vi "Queues vs Local Variables.vi"() -> ()   [LabVIEW 2009]
panel:
  in  "Durée de la boucle (ms)":u16(ring)=50 items=["La même que la boucle productrice"=50, "Vitesse maximale"=0, "2 fois la boucle productrice"=25, "1/2 de la boucle productrice"=100, "1/20 de la boucle productrice"=1000]
  out "Nb de points manqués":i32
  in  "Durée de la boucle (ms)":u16(ring)=50 items=["La même que la boucle productrice"=50, "Vitesse maximale"=0, "2 fois la boucle productrice"=25, "1/2 de la boucle productrice"=100, "1/20 de la boucle productrice"=1000]
  out "Nb d'éléments dans\nla file d'attente":i32(slide) caption="Nb d'éléments dans la file d'attente" scale=0.0..1000.0
  out "Nb de points générés par la boucle productrice":i32
  in  "Stop":bool
  out "Boucle consommatrice de variable locale":dbl(graph)
  out "Boucle consommatrice de file d'attente":dbl(graph)=-9.510565162951542
  out "Boucle productrice":dbl(graph)
  # "Boucle productrice"
  # "Durée de la boucle = 50 ms"
  # "Boucle consommatrice de variable locale"
  # "Boucle consommatrice de file d'attente"
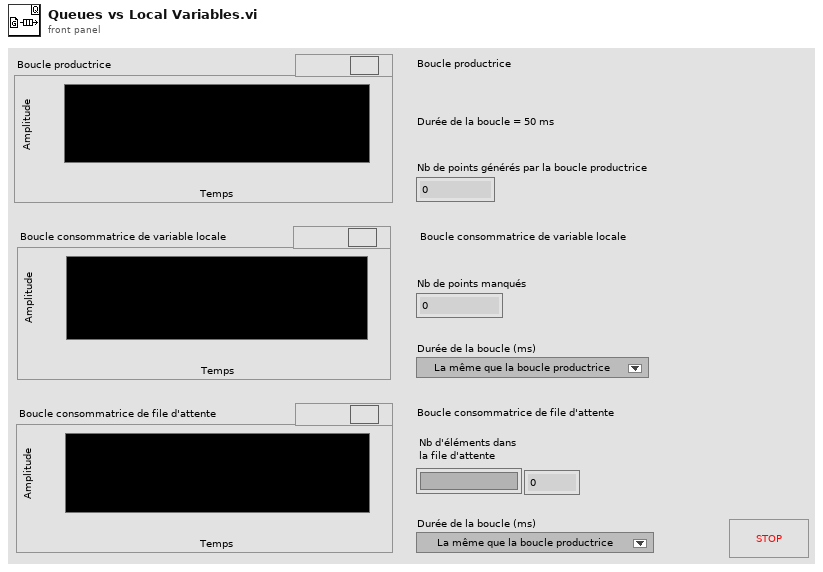
[diagram p1: front panel]
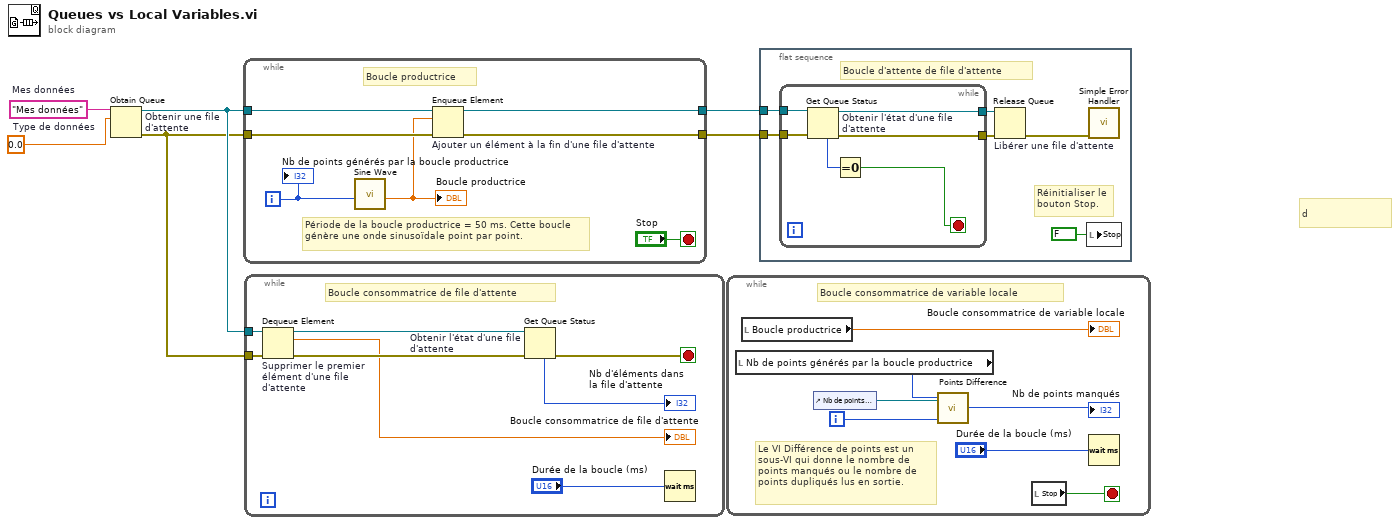
[diagram p0: block diagram]
diagram:
  w5 = "Mes données"  # Mes données
  w6 = 0.0  # Type de données
  # "d"
  n1 = Obtain Queue "Obtenir une file d'attente"(name (unnamed)=w5, element data type=w6) -> (queue out=w4:refnum<queue>, error out=w1:errorcluster)  [unwired: 3 in, 1 out]
  n2 = while {
    tunnel: w4 -> [w11]
    tunnel: w1 -> [w10]
    tunnel: [w8] -> w3
    tunnel: [w7] -> w2
    i -> [w12]
    stop <- "Stop" stop-if-true
    # "Période de la boucle productrice = 50 ms. Cette boucle génère une onde sinusoïdale point par point."
    # "Boucle productrice"
    n3 = call "Sine Wave.vi"("Numérique"=w12) -> ("Signal sinusoïdal"=w9:dbl)  [unwired: 6 out]
    "Boucle productrice" <- w9
    n4 = Enqueue Element "Ajouter un élément à la fin d'une file d'attente"(queue=w11, element=w9, error in (no error)=w10) -> (queue out=w7:refnum<queue>, error out=w8:errorcluster)  [unwired: 2 out]
    "Nb de points générés par la boucle productrice" <- w12
  }
  n5 = while {
    tunnel: w4 -> [w18]
    tunnel: w1 -> [w17]
    stop <- w15 stop-if-true
    # "Boucle consommatrice de file d'attente"
    n6 = Dequeue Element "Supprimer le premier élément d'une file d'attente"(queue=w18, error in (no error)=w17) -> (queue out=w20:refnum<queue>, element=→"Boucle consommatrice de file d'attente":dbl, error out=w19:errorcluster)  [unwired: 2 out]
    n7 = Get Queue Status "Obtenir l'état d'une file d'attente"(queue=w20, error in (no error)=w19) -> (error out=w15:errorcluster, # elements in queue=→"Nb d'éléments dans\nla file d'attente":i32)  [unwired: 7 out]
    n8 = Wait (ms)(milliseconds to wait="Durée de la boucle (ms)") -> ()  [unwired: 1 out]
  }
  n9 = while {
    i -> [w26]
    stop <- w22 stop-if-true
    # "Boucle consommatrice de variable locale"
    # "Le VI Différence de points est un sous-VI qui donne le nombre de points manqués ou le nombre de points dupliqués lus en sortie."
    n10 = local read "Nb de points générés par la boucle productrice"() -> (w27:i32)
    n11 = local read "Boucle productrice"() -> (→"Boucle consommatrice de variable locale":dbl)
    n12 = control-ref of="Nb de points manqués"() -> (w23:refnum<vi>)
    n13 = call "Points Difference.vi"("Nb de points (boucle consommatrice)"=w26, "Refnum de la commande Points manqués"=w23, "Nb de points (boucle productrice)"=w27) -> ("Points manqués"=→"Nb de points manqués":i32)
    n14 = local read "Stop"() -> (w22:bool)
    n15 = Wait (ms)(milliseconds to wait="Durée de la boucle (ms)") -> ()  [unwired: 1 out]
  }
  n16 = flat-sequence {
    tunnel: w3 -> [w31]
    tunnel: w2 -> [w32]
    frame #0 {
      # "Boucle d'attente de file d'attente"
      # "Réinitialiser le \nbouton Stop."
      n17 = while {
        tunnel: w32 -> [w40]
        tunnel: w31 -> [w39]
        tunnel: [w38] -> w30
        tunnel: [w37] -> w29
        stop <- w35 stop-if-true
        n18 = Get Queue Status "Obtenir l'état d'une file d'attente"(queue=w40, error in (no error)=w39) -> (queue out=w37:refnum<queue>, error out=w38:errorcluster, # elements in queue=w36:i32)  [unwired: 6 out]
        n19 = Equal To 0?(x=w36) -> (x = 0?=w35:bool)
      }
      n20 = Release Queue "Libérer une file d'attente"(queue=w29, error in (no error)=w30) -> (error out=w33:errorcluster)  [unwired: 3 out]
      n21 = local write "Stop"(FALSE ("stop")) -> ()
      n22 = call <vilib>:"Simple Error Handler.vi"("error in (no error)"=w33) -> ()  [unwired: 2 in, 7 out]
    }
  }
